vi "Convert with Linear Calibration (inverse) (ND, DBL).vi"(10 "Linear Calibration ND":T1, 11 "A*":T2) -> (3 "A":T2)   [LabVIEW 2011, in "COSYLib.lvlib"]
doc: "Calculates X=(Y-B)/A, with A and B taken from a <B>Linear Calibration</B> cluster."
uses:
  COSYLib.lvlib
  ND Point.ctl
  Linear Calibration ND.ctl
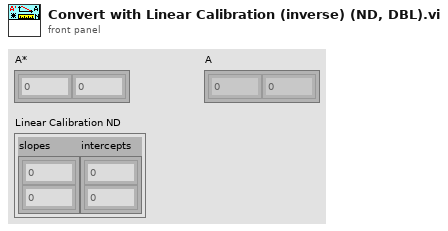
[diagram p1: front panel]
types:
  T1 = typedef "COSYLib.lvlib/Linear Calibration ND.ctl" = cluster{"slopes":dbl[], "intercepts":dbl[]}
  T2 = typedef "COSYLib.lvlib/ND Point.ctl" = dbl[]
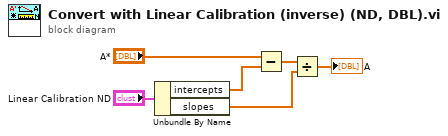
[diagram p0: block diagram]
diagram:
  n1 = Unbundle By Name("Linear Calibration ND") -> ("intercepts"=w4:dbl[], "slopes"=w2:dbl[])
  n2 = Subtract(x="A*", y=w4) -> (x-y=w3:T2)
  n3 = Divide(x=w3, y=w2) -> (x/y=→"A":T2)
